vi "lamp status.vi"(5 "GPIB in":string="18") -> (0 "instrument on":bool, 1 "lamp":T1, 2 "GPIB out":string="18")   [LabVIEW 2015]
uses:
  lamp2.ctl
panel:
  out "powering up":bool
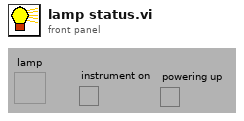
[diagram p1: front panel]
types:
  T1 = typedef "lamp2.ctl" = bool
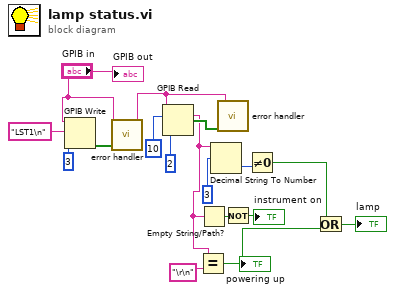
[diagram p0: block diagram]
diagram:
  n1 = GPIB Write(0:"GPIB in", 1:"LST1\n", 2:3) -> (5:w16:bool[])  [unwired: 2 in, 1 out]
  n2 = call "error handler.vi"("status array"=w16, "GPIB in"="GPIB in") -> ("GPIB out"=w8:string)  [unwired: 3 in, 2 out]
  n3 = GPIB Read(0:w8, 1:10, 2:2) -> (5:w4:string, 6:w12:bool[])  [unwired: 2 in, 1 out]
  n4 = Equal?(x=w4, y="\r\n") -> (x = y?=w3:bool)
  "powering up" <- w3
  n5 = Empty String/Path?(string/path=w4) -> (empty?=w7:bool)
  n6 = Decimal String To Number(string=w4, offset=3) -> (number=w10:i32)  [unwired: 1 in, 1 out]
  n7 = call "error handler.vi"("status array"=w12, "GPIB in"=w8) -> ()  [unwired: 3 in, 3 out]
  n8 = Not(x=w7) -> (.not. x?=→"instrument on":bool)
  n9 = Not Equal To 0?(x=w10) -> (x != 0?=w2:bool)
  n10 = Or(x=w2, y=w3) -> (x .or. y?=→"lamp":bool)
  "GPIB out" <- "GPIB in"
